vi "Get Calibration Data for 0 dBm Test Signal.vi"(8 "error in":errorcluster, 11 "Carrier Frequency":dbl format="%#_6p") -> (0 "error out":errorcluster, 3 "Calibration Data":dbl)   [LabVIEW 2017]
uses:
  <vilib>/Utility/file.llb/Read Delimited Spreadsheet (DBL).vi
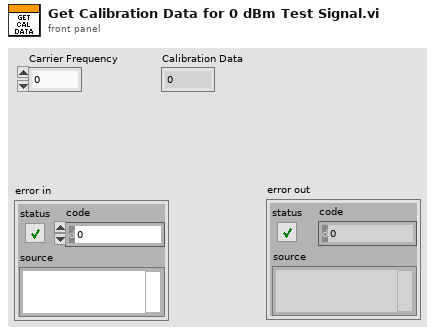
[diagram p1: front panel]
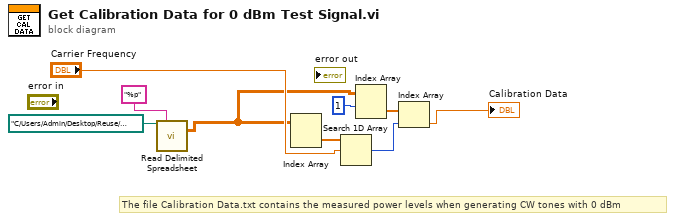
[diagram p0: block diagram]
diagram:
  # "The file Calibration Data.txt contains the measured power levels when generating CW tones with 0 dBm"
  n1 = call-poly <vilib>:"Read Delimited Spreadsheet.vi"("file path (dialog if empty)"=path "C:/Users/Admin/Desktop/Reuse/Scanning Speed PXIe 5668/Calibration Data.txt", "format (%.3f)"="%p") -> ("all rows"=w1:dbl[][])  [unwired: 8 in, 5 out]
  n2 = Index Array(array=w1) -> (element=w4:dbl[])  [unwired: 2 in]
  n3 = Search 1D Array(1D array=w4, element="Carrier Frequency") -> (index of element=w8:i32)  [unwired: 1 in]
  n4 = Index Array(array=w1, index (row)=1) -> (element=w7:dbl[])  [unwired: 1 in]
  n5 = Index Array(array=w7, index=w8) -> (element=→"Calibration Data":dbl)
